vi "4-Wire Register (Boolean array).vi"(0 "data in":bool[](array[boolean])=[FALSE, FALSE, FALSE, FALSE, FALSE, FALSE, FALSE, FALSE, FALSE, FALSE, FALSE, FALSE, FALSE, FALSE, FALSE, FALSE], 2 "reset":bool, 5 "input valid":bool, 12 "ready for output (T)":bool=TRUE) -> (4 "data out":bool[](array[boolean]), 6 "output valid":bool, 14 "ready for input":bool)   [LabVIEW 2018, in "Streaming FPGA.lvlib"]
doc: "Connects two 4-wire handshaking based nodes to each other through a register with cache."
uses:
  Streaming FPGA.lvlib
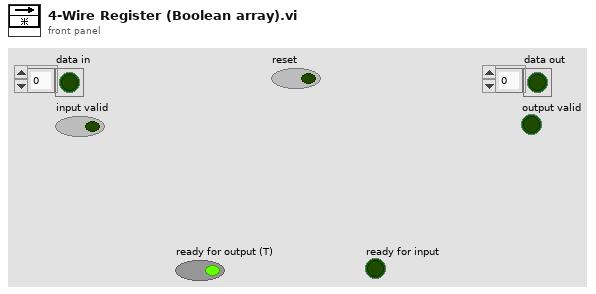
[diagram p1: front panel]
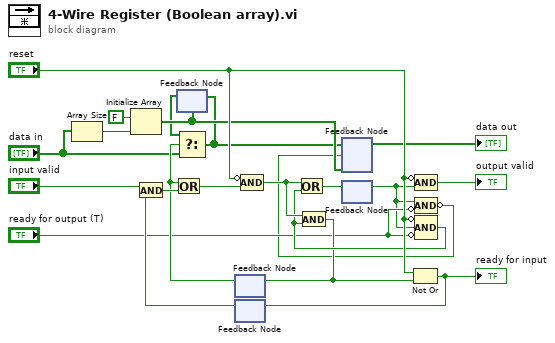
[diagram p0: block diagram]
diagram:
  n1 = Array Size(array="data in") -> (size(s)=w6:i32)
  n2 = Initialize Array(FALSE, w6) -> (w21:bool[])
  n3 = feedback #1(w21) -> (w3:bool[])
  n4 = feedback #2() -> (w16:bool)  [unwired: 1 in]
  n5 = Select(t=w3, s=w16, f="data in") -> (s? t:f=w4:bool[])
  n6 = feedback-in #1(w4) -> ()
  n7 = feedback #3() -> (w14:bool)  [unwired: 1 in]
  n8 = And(x="input valid", y=w14) -> (x .and. y?=w18:bool)
  n9 = Or(x=w16, y=w18) -> (x .or. y?=w13:bool)
  n10 = Compound Arithmetic op=AND(invert "reset", w13) -> (w12:bool)
  n11 = feedback #4(w21) -> (→"data out":bool[])
  n12 = feedback #5() -> (w8:bool)  [unwired: 1 in]
  n13 = Compound Arithmetic op=AND(invert "reset", w8) -> (→"output valid":bool)
  n14 = Compound Arithmetic op=AND(w8, invert "ready for output (T)") -> (invert w7:bool)
  n15 = feedback-in #4(w4, w7) -> ()
  n16 = Compound Arithmetic op=AND(invert "reset", w8, invert "ready for output (T)") -> (w11:bool)
  n17 = Or(x=w12, y=w11) -> (x .or. y?=w19:bool)
  n18 = And(x=w12, y=w11) -> (x .and. y?=w10:bool)
  n19 = feedback-in #2(w10) -> ()
  n20 = feedback-in #5(w19) -> ()
  n21 = Not Or(1:w10, 2:"reset") -> (0:w15:bool)
  "ready for input" <- w15
  n22 = feedback-in #3(w15) -> ()
